vi "CHECK_If_TTL_command_should_be_sent.vi"(2 "Error In":errorcluster, 3 "To be activated in":bool[](array[boolean])) -> (0 "Error Out":errorcluster, 1 "Send a TTL command?":bool[](array[boolean]))   [LabVIEW 2018, in "Tracker.lvlib"]
uses:
  Tracker.lvlib
  <vilib>/ptbypt/NI_PtbyPt.lvlib
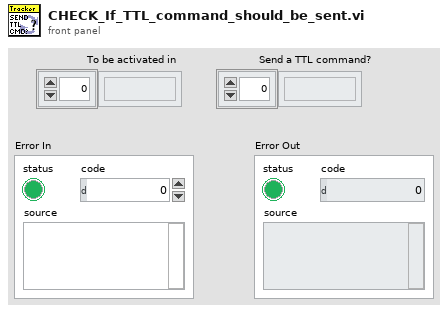
[diagram p1: front panel]
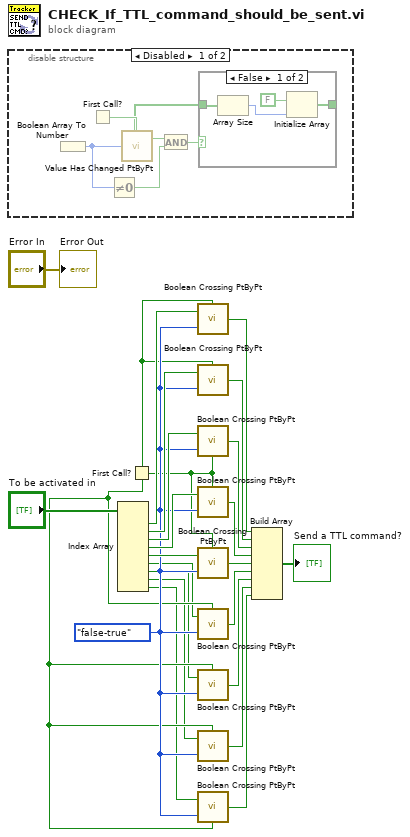
[diagram p0: block diagram]
diagram:
  w10 = enum16{"either", "false-true", "true-false"}."false-true" ("direction")
  n1 = disable-structure shown="Disabled" {
    frame Disabled {
      n2 = First Call?() -> (First Call?: T/F=w29:bool)
      n3 = Boolean Array To Number(Boolean array=w24) -> (number=w28:u32)
      n4 = Not Equal To 0?(x=w28) -> (x != 0?=w27:bool)
      n5 = call <vilib>:"Value Has Changed PtByPt.vi"("input data point"=w28, "initialize"=w29) -> ("has changed"=w26:bool)  [unwired: 1 out]
      n6 = And(x=w26, y=w27) -> (x .and. y?=w25:bool)
      n7 = case shown="False" w25 {
        tunnel: [w30 w34] -> _
        tunnel: [w33 w34] -> w24
        frame False {
          n8 = Array Size(array=w33) -> (size(s)=w32:i32)
          n9 = Initialize Array(FALSE, w32) -> (w30:bool[])
        }
        frame True {
        }
      }
    }
    frame Enabled {
    }
  }
  n10 = Index Array(array="To be activated in") -> (element #1=w22:bool, element #2=w21:bool, element #3=w20:bool, element #4=w19:bool, element #5=w12:bool, element #6=w4:bool, element #7=w3:bool, element #8=w2:bool, element #9=w1:bool)  [unwired: 9 in]
  n11 = First Call?() -> (First Call?: T/F=w5:bool)
  n12 = call <vilib>:"Boolean Crossing PtByPt.vi"("initialize"=w5, "direction"=w10, "input"=w22) -> ("crossing"=w18:bool)
  n13 = call <vilib>:"Boolean Crossing PtByPt.vi"("initialize"=w5, "direction"=w10, "input"=w21) -> ("crossing"=w17:bool)
  n14 = call <vilib>:"Boolean Crossing PtByPt.vi"("initialize"=w5, "direction"=w10, "input"=w20) -> ("crossing"=w16:bool)
  n15 = call <vilib>:"Boolean Crossing PtByPt.vi"("initialize"=w5, "direction"=w10, "input"=w19) -> ("crossing"=w15:bool)
  n16 = call <vilib>:"Boolean Crossing PtByPt.vi"("initialize"=w5, "direction"=w10, "input"=w12) -> ("crossing"=w11:bool)
  n17 = call <vilib>:"Boolean Crossing PtByPt.vi"("initialize"=w5, "direction"=w10, "input"=w4) -> ("crossing"=w9:bool)
  n18 = call <vilib>:"Boolean Crossing PtByPt.vi"("initialize"=w5, "direction"=w10, "input"=w3) -> ("crossing"=w8:bool)
  n19 = call <vilib>:"Boolean Crossing PtByPt.vi"("initialize"=w5, "direction"=w10, "input"=w2) -> ("crossing"=w7:bool)
  n20 = call <vilib>:"Boolean Crossing PtByPt.vi"("initialize"=w5, "direction"=w10, "input"=w1) -> ("crossing"=w6:bool)
  n21 = Build Array(w18, w17, w16, w15, w11, w9, w8, w7, w6) -> (→"Send a TTL command?":bool[])
  "Error Out" <- "Error In"
